vi "_txtData Converter.vi"() -> (0 "Output Text":string)   [LabVIEW 2012]
uses:
  Type/_File Command.ctl
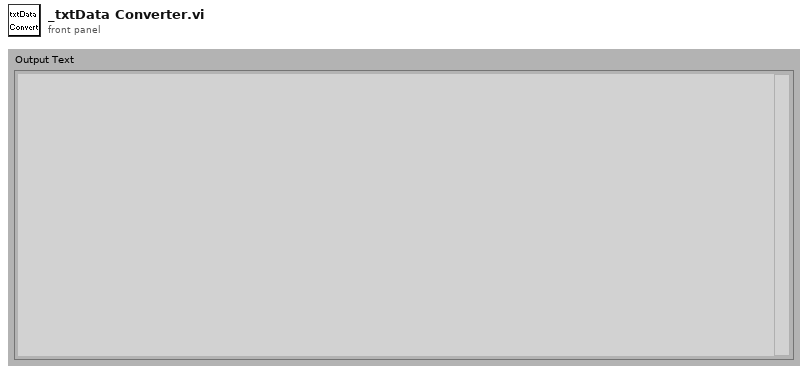
[diagram p1: front panel]
types:
  T1 = enum32{"existing file", "new file", "new or existing file", "existing dir", "new dir", "new or existing dir", "existing file (use LLBs)", "new file (use LLBs)", "new or existing file (use LLBs)", "new or existing file or directory (use LLBs)"}
  T2 = typedef "_File Command.ctl" = enum16{"No Command", "Open", "Open Read", "Write", "Get Spectrum", "Close"}
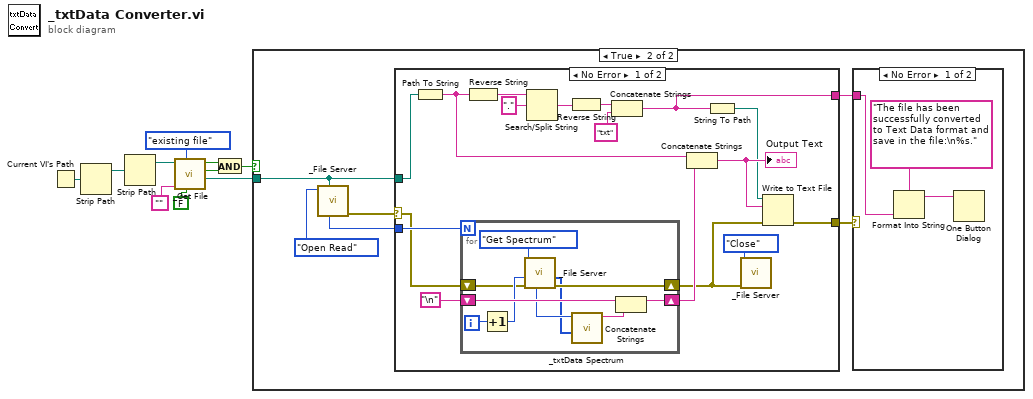
[diagram p0: block diagram]
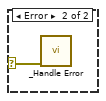
[diagram p3: hidden frame]
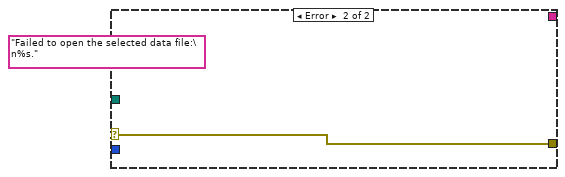
[diagram p4: hidden frame]
diagram:
  n1 = Current VI's Path() -> (path=w7:path)
  n2 = Strip Path(path=w7) -> (stripped path=w8:path)  [unwired: 1 out]
  n3 = Strip Path(path=w8) -> (stripped path=w6:path)  [unwired: 1 out]
  n4 = call "_Get File.vi"("For Write (T)"=FALSE, "select mode (new or existing)"=T1."existing file", "default name"="", "Start Path"=w6) -> ("Seleted File"=w1:path, "Exists"=w3:bool, "Succeeded"=w4:bool)  [unwired: 2 in, 1 out]
  n5 = And(x=w4, y=w3) -> (x .and. y?=w5:bool)
  n6 = case shown="True" w5 {
    tunnel: w1 -> [_ w14]
    frame False {
    }
    frame True {
      n7 = call "_File Server.vi"("file path"=w14, "File Command"=_File_Command."Open Read") -> ("error out"=w15:errorcluster, "Scan# out"=w13:i32)  [unwired: 5 in, 3 out]
      n8 = case shown="No Error" w15 {
        selector: w15 -> [w33 w52]
        tunnel: w14 -> [w35 w51]
        tunnel: [w30 w48] -> w12
        tunnel: w13 -> [w34 _]
        tunnel: [w22 _] -> w11
        frame No Error {
          n9 = Path To String(path=w35) -> (string=w21:string)
          n10 = for {
            N: w34 -> [_]
            shift-right: [w46] -> w37
            shift-left: "\n" -> [w47]
            shift-right: [w41] -> w31
            shift-left: w33 -> [w42]
            i -> [w45]
            n11 = Increment(x=w45) -> (x+1=w43:i32)
            n12 = call "_File Server.vi"("error in (no error)"=w42, "Scan#"=w43, "File Command"=_File_Command."Get Spectrum") -> ("error out"=w41:errorcluster, "Spectrum Out"=w38:u32[], "Scan# out"=w40:i32)  [unwired: 4 in, 2 out]
            n13 = call "_txtData Spectrum.vi"("Spectrum"=w38, "id"=w40) -> ("Output Text"=w39:string)  [unwired: 5 out]
            n14 = Concatenate Strings(w47, w39) -> (w46:string)
          }
          n15 = Reverse String(1:w21) -> (0:w28:string)
          n16 = Search/Split String(string=w28, search string/char (-)=".") -> (match + rest of string=w26:string)  [unwired: 3 out]
          n17 = Reverse String(1:w26) -> (0:w25:string)
          n18 = Concatenate Strings(w25, "txt" ("search string/char (-)")) -> (w22:string)
          n19 = Concatenate Strings(w21, w37) -> (w29:string)
          "Output Text" <- w29
          n20 = String To Path(string=w22) -> (path=w23:path)
          n21 = call "_File Server.vi"("error in (no error)"=w31, "File Command"=_File_Command."Close") -> ()  [unwired: 5 in, 5 out]
          n22 = Write to Text File(file (use dialog)=w23, text=w29, error in=w31) -> (error out=w30:errorcluster)  [unwired: 3 out]
        }
        frame Error {
          n23 = Format Into String(format string="Failed to open the selected data file:\n%s.", w51) -> (resulting string=w49:string)  [unwired: 2 in, 1 out]
          n24 = call "_Construct Error Cluster.vi"("error in"=w52, "reason"=w49) -> ("error out"=w48:errorcluster)  [unwired: 2 in, 3 out]
        }
      }
      n25 = case shown="No Error" w12 {
        selector: w12 -> [_ w20]
        tunnel: w11 -> [w19 _]
        frame No Error {
          n26 = Format Into String(format string="The file has been successfully converted to Text Data format and save in the file:\n%s.", w19) -> (resulting string=w17:string)  [unwired: 2 in, 1 out]
          n27 = One Button Dialog(message=w17) -> ()  [unwired: 2 out]
        }
        frame Error {
          n28 = call "_Handle Error.vi"("error in (no error)"=w20) -> ()  [unwired: 2 in, 5 out]
        }
      }
    }
  }
